vi "Data to txt.vi"(8 "Eixo":string, 9 "2nd column array":dbl[](array[numeric]), 10 "1st column array":dbl[](array[numeric]), 11 "Timestep":string) -> (2 "Data to text file":string)   [LabVIEW 2013]
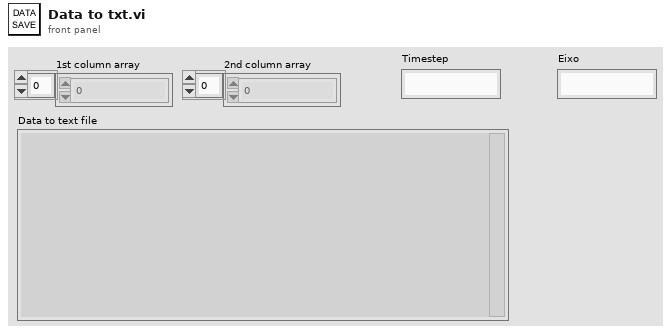
[diagram p1: front panel]
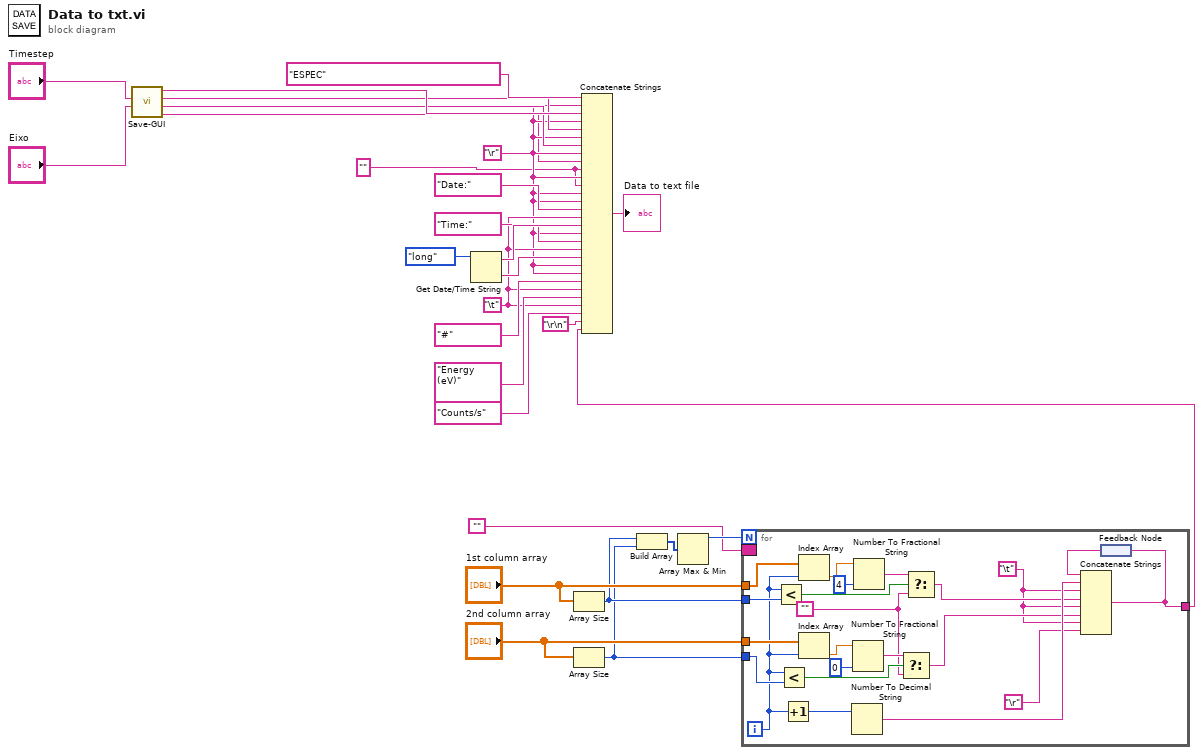
[diagram p0: block diagram]
diagram:
  w3 = "" ("string")
  w13 = "\t"
  w5 = "\r"
  n1 = call "Save-GUI.vi"("Tipo de eixo dos XX"="Eixo", "Time Step:"="Timestep") -> ("Descrição:"=w4:string, "Tipo de eixo dos XX"=w6:string, "Time Step:"=w7:string, "Nome do utilizador:"=w8:string)  [unwired: 4 in]
  n2 = Get Date/Time String(date format (0)=enum16{"short", "long", "abbreviated"}."long") -> (date string=w28:string, time string=w25:string)  [unwired: 2 in]
  n3 = Array Size(array="1st column array") -> (size(s)=w15:i32)
  n4 = Array Size(array="2nd column array") -> (size(s)=w14:i32)
  n5 = Build Array(w15, w14) -> (w22:i32[])
  n6 = Array Max & Min(array=w22) -> (max value=w21:i32)  [unwired: 3 out]
  n7 = for {
    N: w21 -> [_]
    tunnel: "1st column array" -> [w46]
    tunnel: [w49] -> w10
    tunnel: "2nd column array" -> [w48]
    tunnel: w15 -> [w42]
    tunnel: w14 -> [w35]
    border: "" -> [_]
    i -> [w33]
    w31 = ""
    w32 = "\t"
    n8 = Less?(x=w33, y=w42) -> (x < y?=w41:bool)
    n9 = Less?(x=w33, y=w35) -> (x < y?=w34:bool)
    n10 = Increment(x=w33) -> (x+1=w38:i32)
    n11 = Index Array(array=w46, index=w33) -> (element=w43:dbl)
    n12 = Index Array(array=w48, index=w33) -> (element=w47:dbl)
    n13 = Number To Decimal String(number=w38) -> (decimal integer string=w45:string)  [unwired: 1 in]
    n14 = Number To Fractional String(number=w47, precision (6)=i16 0) -> (F-format string=w36:string)  [unwired: 2 in]
    n15 = Number To Fractional String(number=w43, precision (6)=i16 4) -> (F-format string=w40:string)  [unwired: 2 in]
    n16 = Select(t=w36, s=w34, f=w31) -> (s? t:f=w37:string)
    n17 = Select(t=w40, s=w41, f=w31) -> (s? t:f=w39:string)
    n18 = feedback #1() -> (w50:string)
    n19 = Concatenate Strings(w50, w45, w32, w39, w32, w37, w32, "\r") -> (w49:string)
    n20 = feedback-in #1(w49) -> ()
  }
  n21 = Concatenate Strings("ESPEC", w5, w8, w5, w7, w5, w6, w5, w4, w3, w5, w3, w5, w5, "Date:", w13, w28, w5, "Time:", w13, w25, w5, w5, "#", w13, "Energy (eV)", w13, "Counts/s", "\r\n", w10) -> (→"Data to text file":string)
